vi "Get Format Info.vi"(11 "String":string="$AGENT.81,C8.C8,S*03") -> (2 "Format Status":string, 3 "´¹¤ùID":string)   [LabVIEW 2019]
panel:
  in  "ToolString Input":string="$AGENT,53,VS-62U009+VS-69W014*71"
  out "after substring":string
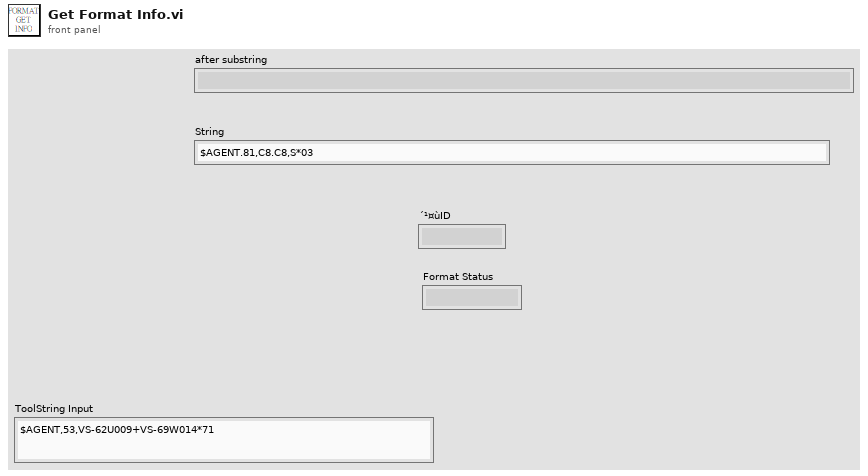
[diagram p1: front panel]
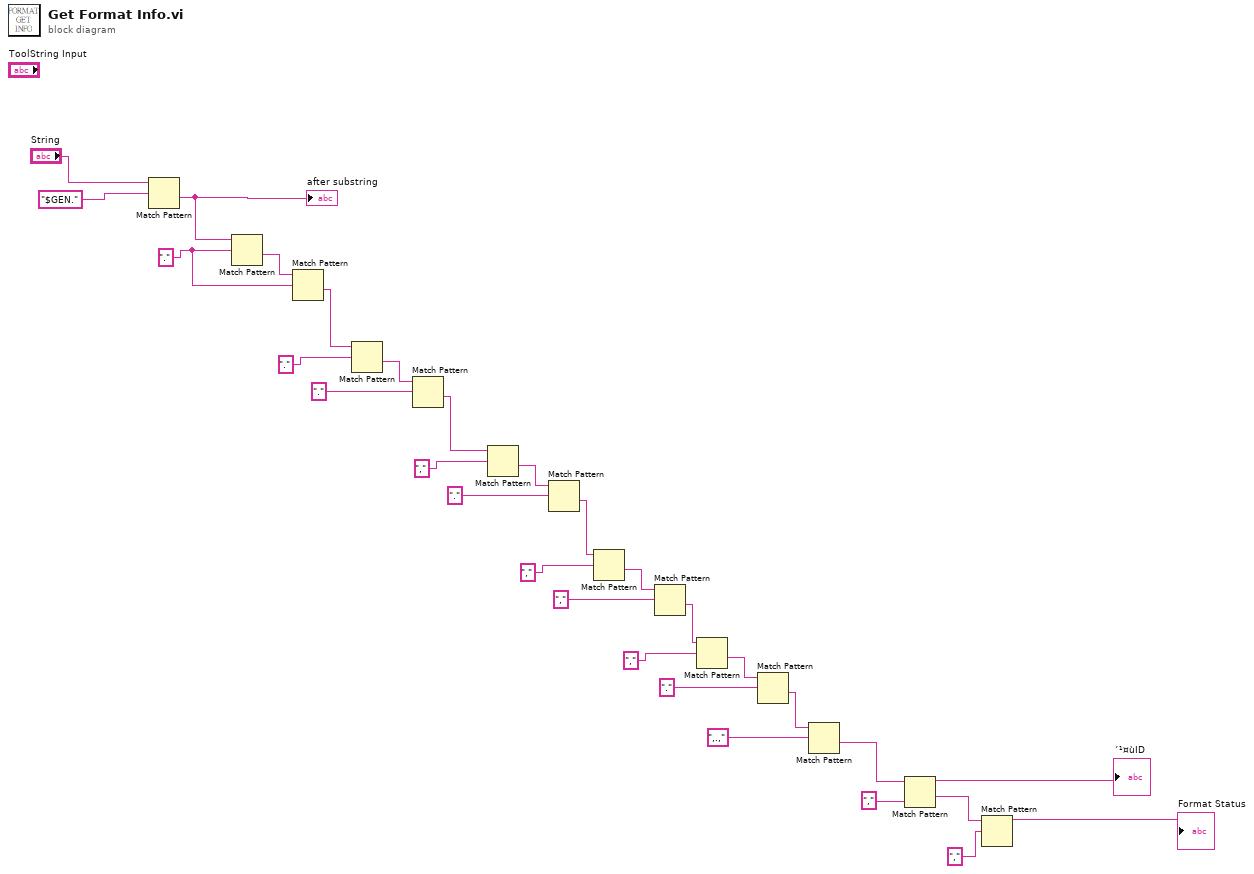
[diagram p0: block diagram]
diagram:
  w26 = "."
  n1 = Match Pattern(string="String", regular expression="$GEN.") -> (after substring=w28:string)  [unwired: 1 in, 3 out]
  "after substring" <- w28
  n2 = Match Pattern(string=w28, regular expression=w26) -> (after substring=w27:string)  [unwired: 1 in, 3 out]
  n3 = Match Pattern(string=w27, regular expression=w26) -> (after substring=w7:string)  [unwired: 1 in, 3 out]
  n4 = Match Pattern(string=w7, regular expression=".") -> (after substring=w23:string)  [unwired: 1 in, 3 out]
  n5 = Match Pattern(string=w23, regular expression=".") -> (after substring=w11:string)  [unwired: 1 in, 3 out]
  n6 = Match Pattern(string=w11, regular expression=",") -> (after substring=w20:string)  [unwired: 1 in, 3 out]
  n7 = Match Pattern(string=w20, regular expression=".") -> (after substring=w10:string)  [unwired: 1 in, 3 out]
  n8 = Match Pattern(string=w10, regular expression=",") -> (after substring=w17:string)  [unwired: 1 in, 3 out]
  n9 = Match Pattern(string=w17, regular expression=",") -> (after substring=w9:string)  [unwired: 1 in, 3 out]
  n10 = Match Pattern(string=w9, regular expression=",") -> (after substring=w14:string)  [unwired: 1 in, 3 out]
  n11 = Match Pattern(string=w14, regular expression=".") -> (after substring=w8:string)  [unwired: 1 in, 3 out]
  n12 = Match Pattern(string=w8, regular expression=",.,") -> (after substring=w5:string)  [unwired: 1 in, 3 out]
  n13 = Match Pattern(string=w5, regular expression=",") -> (before substring=→"´¹¤ùID":string, after substring=w4:string)  [unwired: 1 in, 2 out]
  n14 = Match Pattern(string=w4, regular expression=",") -> (before substring=→"Format Status":string)  [unwired: 1 in, 3 out]
